vi "test Insert Intersection Data In Cluster Array X Correct Y Incorrect.vi"(8 "error in (no error)":errorcluster, 11 "TestCase in":refnum<class "Utility VIs tests.lvclass">) -> (0 "error out":errorcluster, 3 "TestCase out":refnum<class "Utility VIs tests.lvclass">)   [LabVIEW 2014, in "Utility VIs tests.lvclass"]
uses:
  Utility VIs tests.lvclass
  <vilib>/addons/_JKI Toolkits/VI Tester/TestCase.llb/TestCase.lvclass
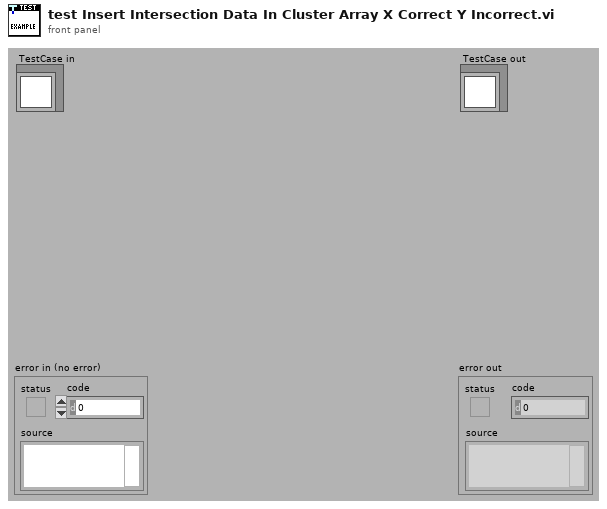
[diagram p1: front panel]
types:
  T1 = cluster{"Time [ms]":dbl, "x":dbl, "y":dbl, "Fout":bool, "Goed":bool}[]
  T2 = cluster{"Time [ms]":dbl, "x":dbl, "y":dbl, "Fout":bool, "Goed":bool}
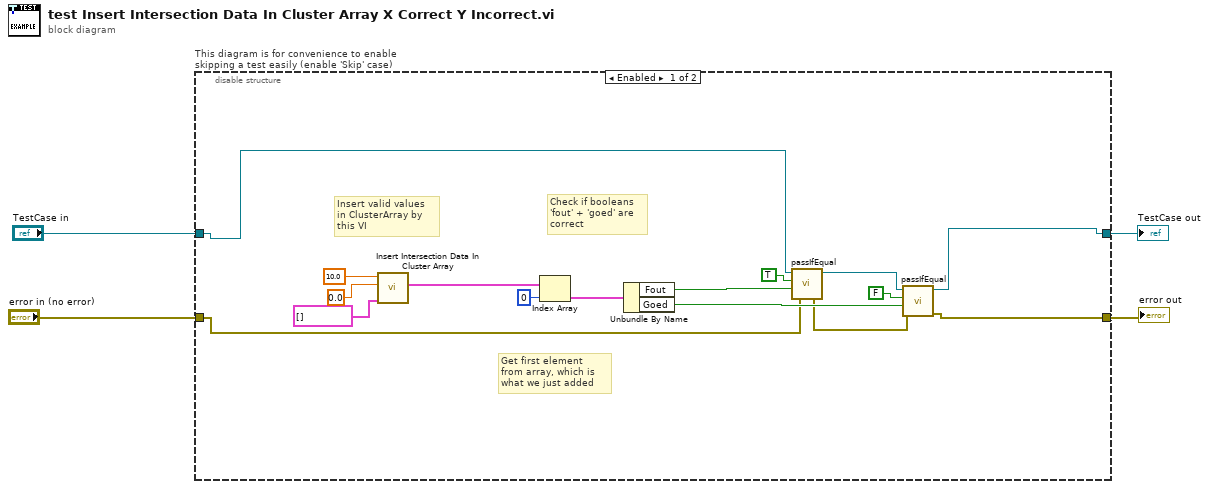
[diagram p0: block diagram]
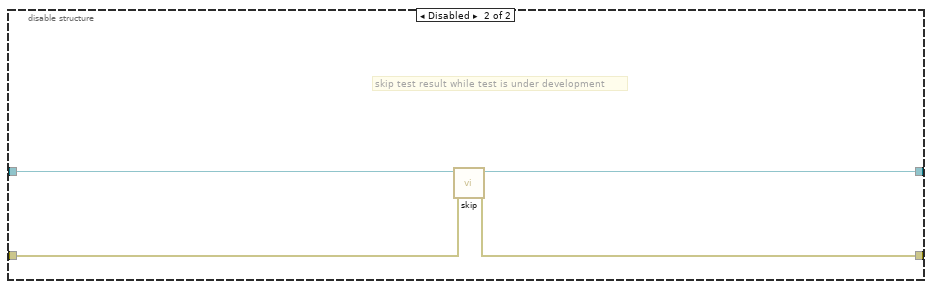
[diagram p2: hidden frame]
diagram:
  n1 = disable-structure "This diagram is for convenience to enable skipping a test easily (enable 'Skip' case)" shown="Enabled" {
    disable-tunnel: "TestCase in" -> [w9 w24]
    disable-tunnel: [w6 w22] -> w1
    disable-tunnel: [w7 w23] -> w3
    disable-tunnel: "error in (no error)" -> [w8 w21]
    frame Enabled {
      # "Get first element\nfrom array, which is \nwhat we just added"
      # "Check if booleans\n'fout' + 'goed' are\ncorrect"
      # "Insert valid values\nin ClusterArray by \nthis VI"
      n2 = call "Insert Intersection Data In Cluster Array.vi"("ClusterArray"=T1 [], "Y"=0.0 ("X"), "X"=10.0) -> ("Intersections"=w18:T1)  [unwired: 8 in]
      n3 = Index Array(array=w18, index=0) -> (element=w16:T2)
      n4 = Unbundle By Name(w16) -> ("Fout"=w15:bool, "Goed"=w14:bool)
      n5 = call-dynamic "passIfEqual.vi"("error in (no error)"=w8, "y"=w15, "x"=TRUE, "TestCase in"=w9) -> ("error out"=w10:errorcluster, "TestCase out"=w11:refnum<class "Utility VIs tests.lvclass">)  [unwired: 6 in]
      n6 = call-dynamic "passIfEqual.vi"("error in (no error)"=w10, "y"=w14, "x"=FALSE, "TestCase in"=w11) -> ("error out"=w7:errorcluster, "TestCase out"=w6:refnum<class "Utility VIs tests.lvclass">)  [unwired: 6 in]
    }
    frame Disabled {
      # "skip test result while test is under development"
      n7 = call <vilib>:"skip.vi"("error in (no error)"=w21, "TestCase in"=w24) -> ("error out"=w23:errorcluster, "TestCase out"=w22:refnum<class "Utility VIs tests.lvclass">)  [unwired: 8 in]
    }
  }
  "error out" <- w3
  "TestCase out" <- w1
